vi "FPGA_Main_Input_Measurement.vi"() -> ()   [LabVIEW 2014]
uses:
  Custom Controls/ActuationControl.ctl
  <vilib>/rvi/Emulation/niFpgaGetClockAttributes.vi
  <vilib>/rvi/Emulation/niFpgaSctlEmulationGetInTimedLoop.vi
  <vilib>/rvi/Emulation/niFpgaEmulationReportErrorSimple.vi
  <vilib>/rvi/Emulation/niFpgaProcessEmulError.vi
  <vilib>/rvi/eio/common/nirviEmuTemplateMethod_errors.vi
  <vilib>/rvi/interface/RandomDataEmulation/niFpgaRandomDataHandleErrors.vi
  <vilib>/rvi/Emulation/niFpgaCriticalErrorInLSC.vi
  <vilib>/eio/EIONode/EIONode.xnode
  <vilib>/rvi/DataTransferAndStorage/Container/XNode/niFpgaContainer.xnode
  <vilib>/rvi/interface/RandomDataEmulation/nirviRandomDataFpgaReadWriteTemplate.vi
  <vilib>/rvi/Analysis/measure/butterworth/XNode/niFpgaButterworthFilter.xnode
panel:
  in  "High Pass?":bool
  in  "Low Pass?":bool
  out "ConnectorB/AO0":u16
  in  "Cluster":T1={"Mode"=enum."Stochastic", "Frequency (Periods/tick)"=0.0024999999441206455, "Phase (period)"=0.0}
  in  "Actuation Period (muS)":u32=5
  in  "Acquisition Period (muS)":u32=2
  in  "stop":bool
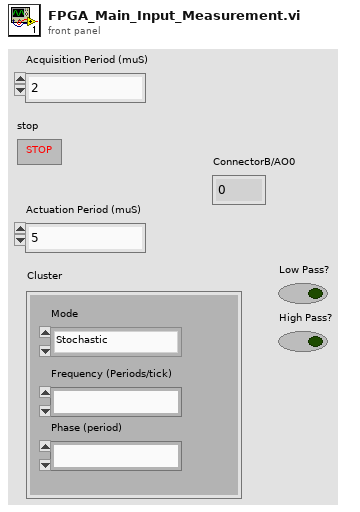
[diagram p1: front panel]
types:
  T1 = typedef "ActuationControl.ctl" = cluster{"Mode":enum16{"Square Wave", "Sine Wave", "White Noise", "Stochastic"}, "Frequency (Periods/tick)":fxp<+,32,0>, "Phase (period)":fxp<+,32,0>}
  T2 = enum16{"Square Wave", "Sine Wave", "White Noise", "Stochastic"}
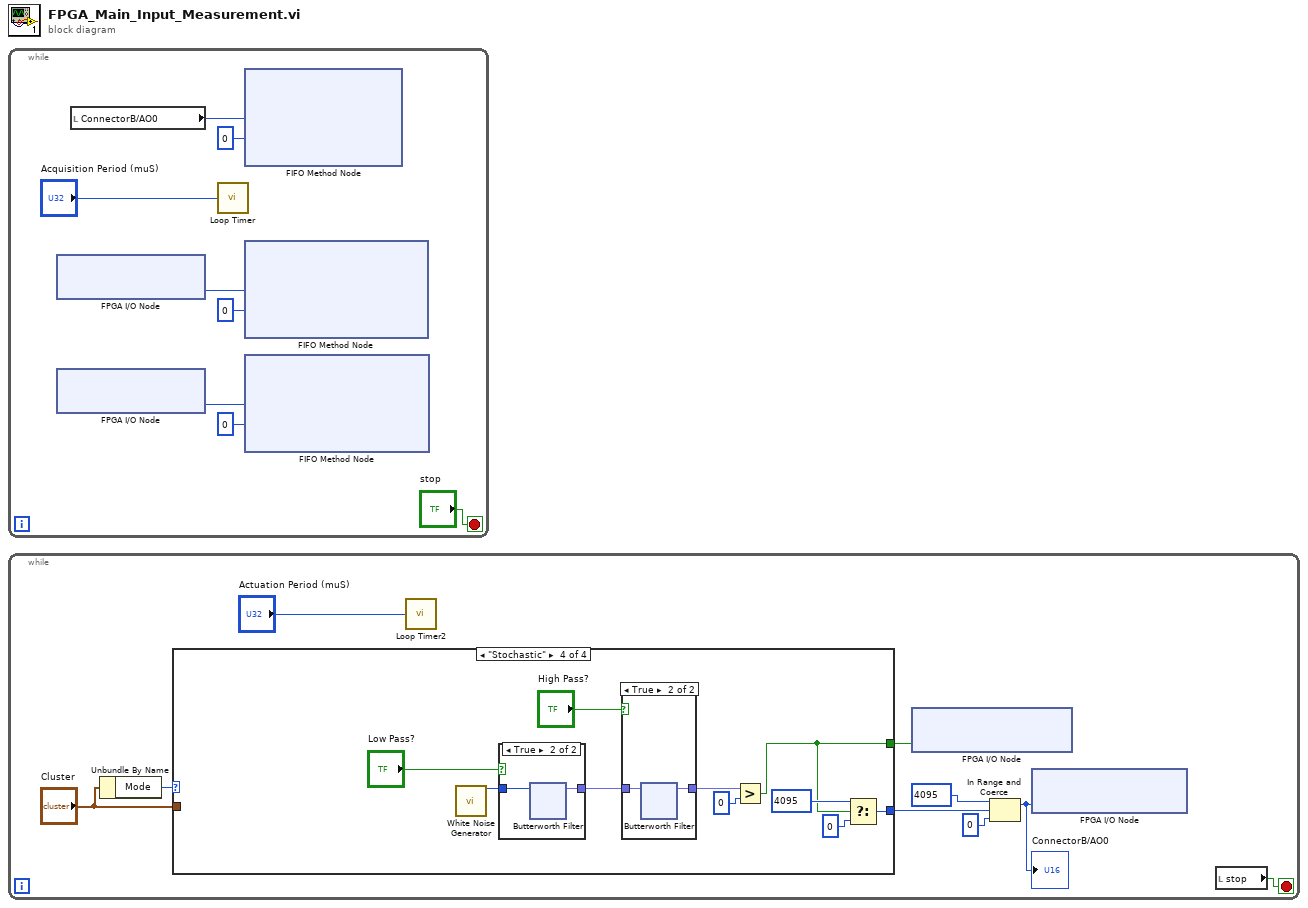
[diagram p0: block diagram]
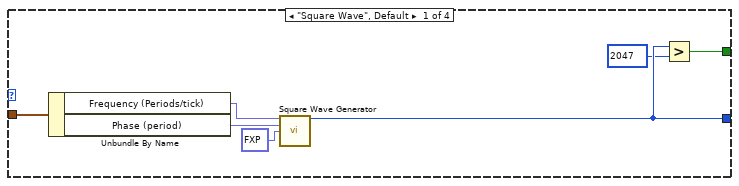
[diagram p2: hidden frame]
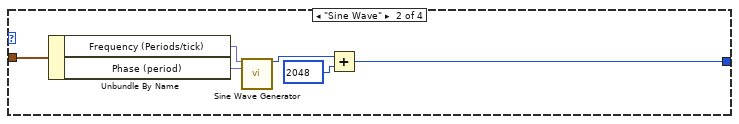
[diagram p3: hidden frame]
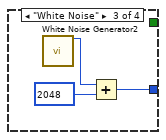
[diagram p4: hidden frame]
diagram:
  n1 = while {
    stop <- "stop" stop-if-true
    n2 = xnode "FPGA I/O Node"() -> ("ConnectorB/AI0"=w7:u16)  [unwired: 1 in, 1 out]
    n3 = xnode "FPGA I/O Node"() -> ("ConnectorC/AI0"=w2:i16)  [unwired: 1 in, 1 out]
    n4 = local read "ConnectorB/AO0"() -> (w4:u16)
    n5 = call "Loop Timer"("Count(uSec)"="Acquisition Period (muS)") -> ()  [unwired: 1 out]
    n6 = xnode ("FIFO Method Node")("Element"=w4, "Timeout"=0) -> ()  [unwired: 1 in, 2 out]
    n7 = xnode ("FIFO Method Node")("Element"=w7, "Timeout"=0) -> ()  [unwired: 1 in, 2 out]
    n8 = xnode ("FIFO Method Node")("Element"=w2, "Timeout"=0) -> ()  [unwired: 1 in, 2 out]
  }
  n9 = while {
    stop <- w16 stop-if-true
    n10 = Unbundle By Name("Cluster") -> ("Mode"=w15:T2)
    n11 = case shown="\"Stochastic\"" w15 {
      tunnel: "Cluster" -> [w24 w27 _ _]
      tunnel: [w20 w29 w31 w40] -> w10
      tunnel: [w18 _ _ w39] -> w9
      frame "Square Wave", Default {
        n12 = Unbundle By Name(w24) -> ("Frequency (Periods/tick)"=w23:fxp<+,32,0>, "Phase (period)"=w22:fxp<+,32,0>)
        n13 = call "Square Wave Generator"("frequency (periods/tick)"=w23, "phase offset (periods)"=w22, "duty cycle (periods)"=fxp<+,32,0> 0.5) -> ("square wave out"=w20:i16)  [unwired: 12 in]
        n14 = Greater?(x=w20, y=i16 2047) -> (0:w18:bool)
      }
      frame "Sine Wave" {
        n15 = Unbundle By Name(w27) -> ("Frequency (Periods/tick)"=w26:fxp<+,32,0>, "Phase (period)"=w25:fxp<+,32,0>)
        n16 = call "Sine Wave Generator"("frequency (periods/tick)"=w26, "phase offset (periods)"=w25) -> ("sine out"=w30:i16)  [unwired: 13 in]
        n17 = Add(x=w30, y=i16 2048) -> (x+y=w29:i16)
      }
      frame "White Noise" {
        n18 = call "White Noise Generator2"() -> ("white noise out"=w32:i16)  [unwired: 15 in]
        n19 = Add(x=w32, y=i16 2048) -> (x+y=w31:i16)
      }
      frame "Stochastic" {
        n20 = call "White Noise Generator"() -> ("white noise out"=w37:i16)  [unwired: 15 in]
        n21 = case shown="True" "Low Pass?" {
          tunnel: w37 -> [w54 w56]
          tunnel: [w54 w55] -> w35
          frame False {
          }
          frame True {
            n22 = xnode "Butterworth Filter"("input data"=w56) -> ("output data"=w55:fxp<+/-,20,20>)  [unwired: 2 in]
          }
        }
        n23 = case shown="True" "High Pass?" {
          tunnel: w35 -> [w44 w46]
          tunnel: [w44 w45] -> w34
          frame False {
          }
          frame True {
            n24 = xnode "Butterworth Filter"("input data"=w46) -> ("output data"=w45:fxp<+/-,24,24>)  [unwired: 2 in]
          }
        }
        n25 = Greater?(x=w34, y=i16 0) -> (0:w39:bool)
        n26 = Select(t=u16 4095 ("y"), s=w39, f=u16 0 ("lower limit")) -> (s? t:f=w40:u16)
      }
    }
    n27 = call "Loop Timer2"("Count(uSec)"="Actuation Period (muS)") -> ()  [unwired: 1 out]
    n28 = xnode "FPGA I/O Node"("ConnectorB/DIO0"=w9) -> ()  [unwired: 1 in, 1 out]
    n29 = In Range and Coerce(upper limit=u16 4095 ("y"), x=w10, lower limit=u16 0) -> (coerced(x)=w11:u16)  [unwired: 1 out]
    "ConnectorB/AO0" <- w11
    n30 = xnode "FPGA I/O Node"("ConnectorB/AO0"=w11) -> ()  [unwired: 1 in, 1 out]
    n31 = local read "stop"() -> (w16:bool)
  }
